vi "traj_coe_write_CPT_final.vi"() -> ()   [LabVIEW 2014]
uses:
  <vilib>/Utility/file.llb/Read From Spreadsheet File (DBL).vi
  <vilib>/FPGAPlugInAG/cRIO-9066/niLvFpga_Open_cRIO-9066.vi
  <vilib>/Utility/error.llb/Error Cluster From Error Code.vi
  <vilib>/rvi/errors/niLvFpgaAdjustHostInterfaceError.vi
  <vilib>/rvi/interface/nirviOpenFPGA/nirviOpenFPGA.xnode
  FPGA Bitfiles/forcecontroledu_FPGATarget_forcecontrolfric_QscRzYavH1A.lvbitx
  FPGA VIs/force_control_friction_model_final_twomotor_vstiff_imp_newdio_newfric_new_edu.vi
  <vilib>/rvi/interface/nirviMethod/nirviMethod.xnode
  <vilib>/FPGAPlugInAG/cRIO-9066/niLvFpga_WriteFifo_cRIO-9066.vi
  <vilib>/rvi/errors/niLvFpgaMergeErrorWithErrorCode.vi
panel:
  out "A3":dbl[](array[numeric]) format="%.2f"
  out "writing_done":bool
  in  "stop":bool
  out "A1":dbl[](array[numeric]) format="%.2f"
  out "A2":dbl[](array[numeric]) format="%.2f"
  out "A0":dbl[](array[numeric]) format="%.2f"
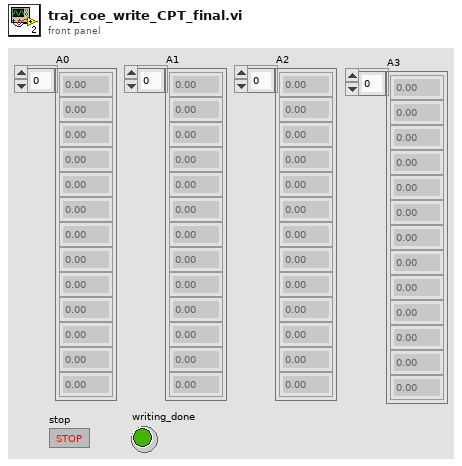
[diagram p1: front panel]
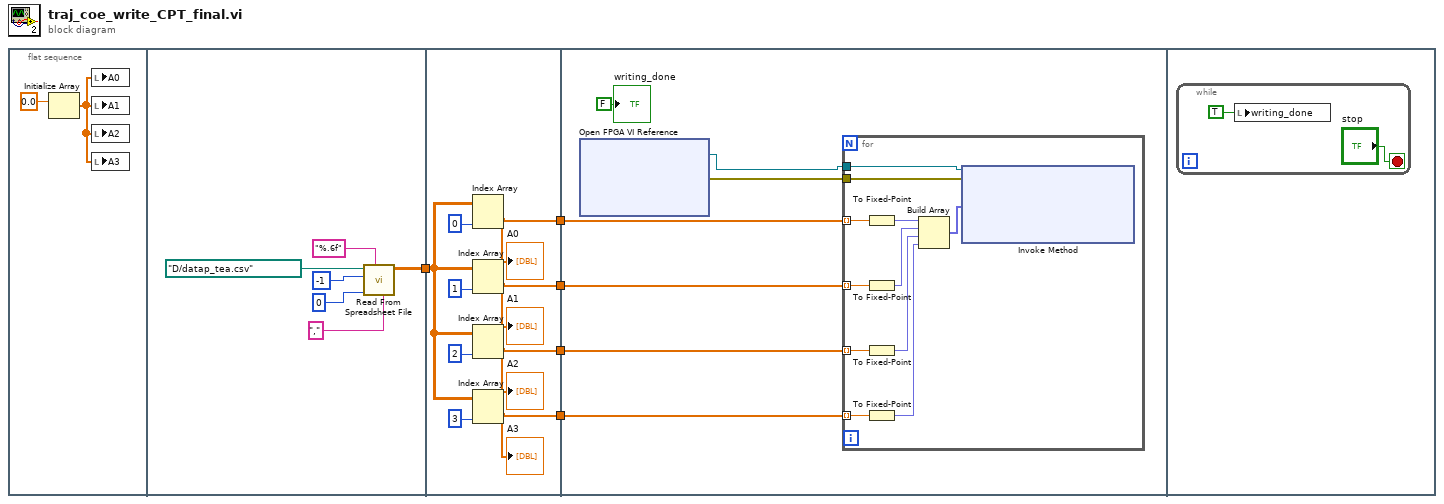
[diagram p0: block diagram]
diagram:
  n1 = flat-sequence {
    tunnel: [w8] -> w5
    tunnel: w5 -> [w15]
    tunnel: [w19] -> w4
    tunnel: [w18] -> w3
    tunnel: [w17] -> w2
    tunnel: [w14] -> w1
    tunnel: w4 -> [w29]
    tunnel: w3 -> [w28]
    tunnel: w2 -> [w27]
    tunnel: w1 -> [w25]
    frame #0 {
      n2 = Initialize Array(0.0 ("element")) -> (w6:dbl[])  [unwired: 1 in]
      n3 = local write "A0"(w6) -> ()
      n4 = local write "A1"(w6) -> ()
      n5 = local write "A2"(w6) -> ()
      n6 = local write "A3"(w6) -> ()
    }
    frame #1 {
      n7 = call-poly <vilib>:"Read From Spreadsheet File.vi"("delimiter (\\t)"="," ("delimiter (\\t)"), "format (%.3f)"="%.6f" ("format (%d)"), "max characters/row  (no limit:0)"=0, "number of rows (all:-1)"=-1, "file path (dialog if empty)"=path "D:/datap_tea.csv") -> ("all rows"=w8:dbl[][])  [unwired: 2 in, 4 out]
    }
    frame #2 {
      n8 = Index Array(array=w15, index (col)=0 ("disabled index (col)")) -> (element=w19:dbl[])  [unwired: 1 in]
      "A0" <- w19
      n9 = Index Array(array=w15, index (col)=1 ("disabled index (col)")) -> (element=w18:dbl[])  [unwired: 1 in]
      "A1" <- w18
      n10 = Index Array(array=w15, index (col)=2 ("disabled index (col)")) -> (element=w17:dbl[])  [unwired: 1 in]
      "A2" <- w17
      n11 = Index Array(array=w15, index (col)=3 ("disabled index (col)")) -> (element=w14:dbl[])  [unwired: 1 in]
      "A3" <- w14
    }
    frame #3 {
      n12 = xnode "Open FPGA VI Reference"() -> ("FPGA VI Reference Out"=w24:refnum<k20>, "error out"=w23:errorcluster)  [unwired: 2 in]
      n13 = for {
        tunnel: w24 -> [w32]
        tunnel: w23 -> [w31]
        tunnel: w29 -> [w40] mode=indexing
        tunnel: w28 -> [w39] mode=indexing
        tunnel: w27 -> [w38] mode=indexing
        tunnel: w25 -> [w34] mode=indexing
        n14 = To Fixed-Point(number=w40) -> (fixed-point=w37:fxp<+/-,30,15>)  [unwired: 1 in]
        n15 = To Fixed-Point(number=w39) -> (fixed-point=w36:fxp<+/-,30,15>)  [unwired: 1 in]
        n16 = To Fixed-Point(number=w38) -> (fixed-point=w35:fxp<+/-,30,15>)  [unwired: 1 in]
        n17 = To Fixed-Point(number=w34) -> (fixed-point=w33:fxp<+/-,30,15>)  [unwired: 1 in]
        n18 = Build Array(w37, w36, w35, w33) -> (w30:fxp<+/-,30,15>[])
        n19 = xnode "Invoke Method"("FPGA VI Reference In"=w32, "error in"=w31, "Data"=w30) -> ()  [unwired: 1 in, 3 out]
      }
      "writing_done" <- FALSE ("writing_done")
    }
    frame #4 {
      n20 = while {
        stop <- "stop" stop-if-true
        n21 = local write "writing_done"(TRUE ("writing_done")) -> ()
      }
    }
  }
